vi "softmax_sub.vi"(1 "Input":ext[](array[numeric])) -> (0 "Output":ext[](array[numeric]))   [LabVIEW 2021]
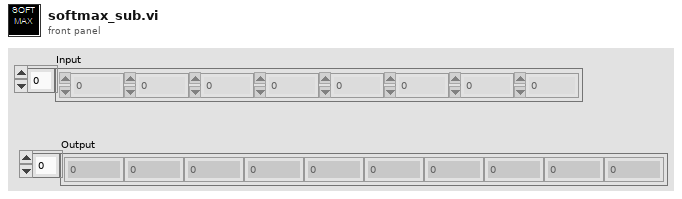
[diagram p1: front panel]
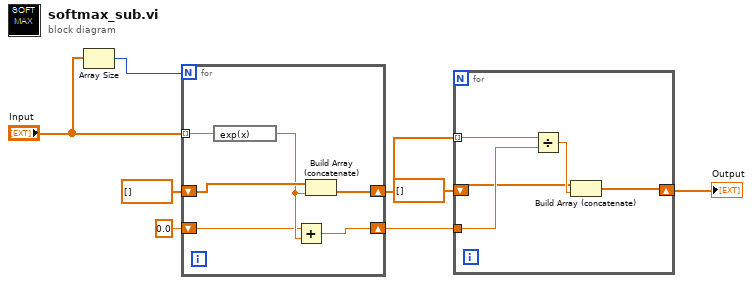
[diagram p0: block diagram]
diagram:
  n1 = Array Size(array="Input") -> (size(s)=w6:i32)
  n2 = for {
    N: w6 -> [_]
    tunnel: "Input" -> [w14] mode=indexing
    shift-right: [w13] -> w3
    shift-left: dbl[] [] -> [w12]
    shift-right: [w11] -> w4
    shift-left: 0.0 -> [w9]
    n3 = expression code="exp(x)"(w14) -> (w10:ext)
    n4 = Add(x=w9, y=w10) -> (x+y=w11:ext)
    n5 = Build Array (concatenate)(w12, w10) -> (w13:ext[])
  }
  n6 = for {
    tunnel: w3 -> [w19] mode=indexing
    tunnel: w4 -> [w18]
    shift-right: [w17] -> w1
    shift-left: dbl[] [] -> [w15]
    n7 = Divide(x=w19, y=w18) -> (x/y=w16:ext)
    n8 = Build Array (concatenate)(w15, w16) -> (w17:ext[])
  }
  "Output" <- w1
